vi "Base Attributes.vi"(4 "Application Ref":refnum<vi>, 5 "UID":string, 6 "Actor Ref":refnum<vi>, 7 "Address":refnum<user-event>, 9 "Unified Msg Set":T1, 10 "Event Ref":refnum<event-registration>) -> (2 "Attributes":refnum<class "Attributes.lvclass">)   [LabVIEW 2025, in "jettl.lvlib" / "Attributes.lvlib"]
uses:
  Attributes.lvlib
  Attributes/Attributes.lvclass
  Msg/Msg.lvclass
  Actor/Msg Set.ctl
  Base Attributes/Base Attributes.lvclass
  C:/git/jettl/src/jettl/jettl/Attributes/Attributes/Attributes.lvclass
  Actor/Actor.lvlib
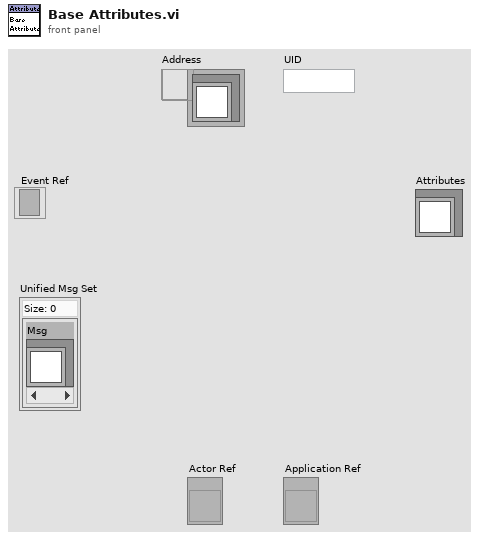
[diagram p1: front panel]
types:
  T1 = typedef "jettl.lvlib/Actor.lvlib/Msg Set.ctl" = set{refnum<class "Msg.lvclass">}
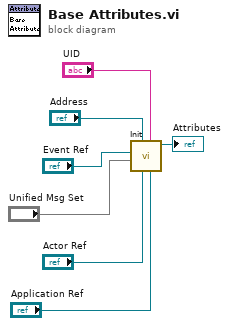
[diagram p0: block diagram]
diagram:
  n1 = call "Init.vi"("Application Ref"="Application Ref", "UID"="UID", "Actor Ref"="Actor Ref", "Address"="Address", "Unified Msg Set"="Unified Msg Set", "Event Ref"="Event Ref") -> ("Base Attributes out"=→"Attributes":refnum<class "Base Attributes.lvclass">)  [unwired: 5 in]
